vi "VI Tree.vi"   [LabVIEW 2012, in "Agilent ESG Series.lvlib"]
doc: "This is the instrument driver for the Hewlett Packard ESG/ESG-D Series Signal Generator. The VI Tree displays all the user-callable VIs of the instrument driver in an organized table.\n\n\nThis VI Tree contains all of the VI's in the LabVIEW template driver. These VI's are intended to be used as starting points for creating your own driver VIs for a particular instrument."
uses:
  <instrlib>/Agilent ESG Series/Agilent ESG Series.lvlib
panel:
  # "(c) 2005 - 2013 National Instruments.  ALL RIGHTS RESERVED."
  # "SEE DIAGRAM\nFOR VI TREE."
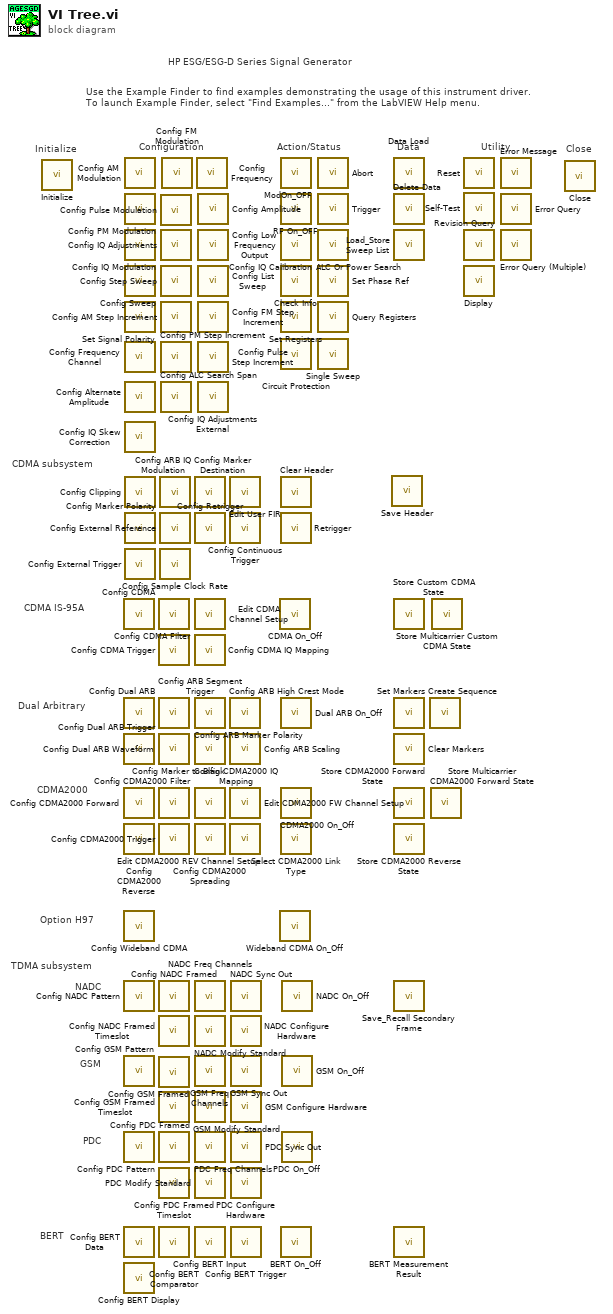
[diagram p0: block diagram]
diagram:
  # "HP ESG/ESG-D Series Signal Generator"
  # "CDMA2000"
  # "TDMA subsystem"
  # "CDMA subsystem"
  # "BERT"
  # "Option H97"
  # "Dual Arbitrary"
  # "CDMA IS-95A"
  # "PDC"
  # "GSM"
  # "NADC"
  # "Use the Example Finder to find examples demonstrating the usage of this instrument driver.\nTo launch Example Finder, select \"Find Examples...\" from the LabVIEW Help menu."
  # "Configuration"
  # "Utility"
  # "Data"
  # "Action/Status"
  # "Close"
  # "Initialize"
  n1 = call <instrlib>:"Initialize.vi"() -> ()  [unwired: 14 in, 2 out]
  n2 = call <instrlib>:"Config CDMA.vi"() -> ()  [unwired: 18 in, 2 out]
  n3 = call <instrlib>:"Config Dual ARB.vi"() -> ()  [unwired: 14 in, 2 out]
  n4 = call <instrlib>:"Config Dual ARB Trigger.vi"() -> ()  [unwired: 14 in, 2 out]
  n5 = call <instrlib>:"Config CDMA2000 Forward.vi"() -> ()  [unwired: 18 in, 2 out]
  n6 = call <instrlib>:"Config CDMA2000 Reverse.vi"() -> ()  [unwired: 18 in, 2 out]
  n7 = call <instrlib>:"Config Wideband CDMA.vi"() -> ()  [unwired: 14 in, 2 out]
  n8 = call <instrlib>:"Config NADC Pattern.vi"() -> ()  [unwired: 14 in, 2 out]
  n9 = call <instrlib>:"Config GSM Pattern.vi"() -> ()  [unwired: 14 in, 2 out]
  n10 = call <instrlib>:"Config PDC Pattern.vi"() -> ()  [unwired: 14 in, 2 out]
  n11 = call <instrlib>:"Config BERT Data.vi"() -> ()  [unwired: 18 in, 2 out]
  n12 = call <instrlib>:"Config BERT Display.vi"() -> ()  [unwired: 10 in, 2 out]
  n13 = call <instrlib>:"Config AM Modulation.vi"() -> ()  [unwired: 18 in, 2 out]
  n14 = call <instrlib>:"Config PM Modulation.vi"() -> ()  [unwired: 18 in, 2 out]
  n15 = call <instrlib>:"Config IQ Modulation.vi"() -> ()  [unwired: 14 in, 2 out]
  n16 = call <instrlib>:"Config Sweep.vi"() -> ()  [unwired: 18 in, 2 out]
  n17 = call <instrlib>:"Set Signal Polarity.vi"() -> ()  [unwired: 10 in, 2 out]
  n18 = call <instrlib>:"Config Frequency Channel.vi"() -> ()  [unwired: 14 in, 2 out]
  n19 = call <instrlib>:"Config Alternate Amplitude.vi"() -> ()  [unwired: 18 in, 2 out]
  n20 = call <instrlib>:"Config IQ Skew Correction.vi"() -> ()  [unwired: 14 in, 2 out]
  n21 = call <instrlib>:"Config Clipping.vi"() -> ()  [unwired: 18 in, 2 out]
  n22 = call <instrlib>:"Config Marker Polarity.vi"() -> ()  [unwired: 18 in, 2 out]
  n23 = call <instrlib>:"Config External Trigger.vi"() -> ()  [unwired: 14 in, 2 out]
  n24 = call <instrlib>:"Config CDMA Filter.vi"() -> ()  [unwired: 14 in, 2 out]
  n25 = call <instrlib>:"Config CDMA Trigger.vi"() -> ()  [unwired: 14 in, 2 out]
  n26 = call <instrlib>:"Config ARB Segment Trigger.vi"() -> ()  [unwired: 14 in, 2 out]
  n27 = call <instrlib>:"Config Dual ARB Waveform.vi"() -> ()  [unwired: 18 in, 2 out]
  n28 = call <instrlib>:"Config CDMA2000 Filter.vi"() -> ()  [unwired: 14 in, 2 out]
  n29 = call <instrlib>:"Config CDMA2000 Trigger.vi"() -> ()  [unwired: 14 in, 2 out]
  n30 = call <instrlib>:"Config NADC Framed.vi"() -> ()  [unwired: 14 in, 2 out]
  n31 = call <instrlib>:"Config NADC Framed Timeslot.vi"() -> ()  [unwired: 14 in, 2 out]
  n32 = call <instrlib>:"Config GSM Framed.vi"() -> ()  [unwired: 14 in, 2 out]
  n33 = call <instrlib>:"Config GSM Framed Timeslot.vi"() -> ()  [unwired: 18 in, 2 out]
  n34 = call <instrlib>:"Config PDC Framed.vi"() -> ()  [unwired: 14 in, 2 out]
  n35 = call <instrlib>:"Config PDC Framed Timeslot.vi"() -> ()  [unwired: 14 in, 2 out]
  n36 = call <instrlib>:"Config BERT Comparator.vi"() -> ()  [unwired: 10 in, 2 out]
  n37 = call <instrlib>:"Config ARB IQ Modulation.vi"() -> ()  [unwired: 14 in, 2 out]
  n38 = call <instrlib>:"Config External Reference.vi"() -> ()  [unwired: 18 in, 2 out]
  n39 = call <instrlib>:"Config Sample Clock Rate.vi"() -> ()  [unwired: 14 in, 2 out]
  n40 = call <instrlib>:"Config Pulse Modulation.vi"() -> ()  [unwired: 14 in, 2 out]
  n41 = call <instrlib>:"Config IQ Adjustments.vi"() -> ()  [unwired: 14 in, 2 out]
  n42 = call <instrlib>:"Config Step Sweep.vi"() -> ()  [unwired: 14 in, 2 out]
  n43 = call <instrlib>:"Config AM Step Increment.vi"() -> ()  [unwired: 14 in, 2 out]
  n44 = call <instrlib>:"Config PM Step Increment.vi"() -> ()  [unwired: 14 in, 2 out]
  n45 = call <instrlib>:"Config ALC Search Span.vi"() -> ()  [unwired: 18 in, 2 out]
  n46 = call <instrlib>:"Config FM Modulation.vi"() -> ()  [unwired: 18 in, 2 out]
  n47 = call <instrlib>:"Config Marker Destination.vi"() -> ()  [unwired: 18 in, 2 out]
  n48 = call <instrlib>:"Config Retrigger.vi"() -> ()  [unwired: 14 in, 2 out]
  n49 = call <instrlib>:"Edit CDMA Channel Setup.vi"() -> ()  [unwired: 14 in, 2 out]
  n50 = call <instrlib>:"Config CDMA IQ Mapping.vi"() -> ()  [unwired: 14 in, 2 out]
  n51 = call <instrlib>:"Config ARB Marker Polarity.vi"() -> ()  [unwired: 14 in, 2 out]
  n52 = call <instrlib>:"Config Marker to Blank.vi"() -> ()  [unwired: 14 in, 2 out]
  n53 = call <instrlib>:"Config CDMA2000 IQ Mapping.vi"() -> ()  [unwired: 14 in, 2 out]
  n54 = call <instrlib>:"Config CDMA2000 Spreading.vi"() -> ()  [unwired: 14 in, 2 out]
  n55 = call <instrlib>:"NADC Freq Channels.vi"() -> ()  [unwired: 10 in, 2 out]
  n56 = call <instrlib>:"NADC Modify Standard.vi"() -> ()  [unwired: 14 in, 2 out]
  n57 = call <instrlib>:"GSM Freq Channels.vi"() -> ()  [unwired: 10 in, 2 out]
  n58 = call <instrlib>:"GSM Modify Standard.vi"() -> ()  [unwired: 14 in, 2 out]
  n59 = call <instrlib>:"PDC Freq Channels.vi"() -> ()  [unwired: 10 in, 2 out]
  n60 = call <instrlib>:"PDC Modify Standard.vi"() -> ()  [unwired: 14 in, 2 out]
  n61 = call <instrlib>:"Config BERT Input.vi"() -> ()  [unwired: 14 in, 2 out]
  n62 = call <instrlib>:"Config Frequency.vi"() -> ()  [unwired: 14 in, 2 out]
  n63 = call <instrlib>:"Config Amplitude.vi"() -> ()  [unwired: 14 in, 2 out]
  n64 = call <instrlib>:"Config Low Frequency Output.vi"() -> ()  [unwired: 14 in, 2 out]
  n65 = call <instrlib>:"Config List Sweep.vi"() -> ()  [unwired: 14 in, 2 out]
  n66 = call <instrlib>:"Config FM Step Increment.vi"() -> ()  [unwired: 14 in, 2 out]
  n67 = call <instrlib>:"Config Pulse Step Increment.vi"() -> ()  [unwired: 14 in, 2 out]
  n68 = call <instrlib>:"Config IQ Adjustments External.vi"() -> ()  [unwired: 14 in, 2 out]
  n69 = call <instrlib>:"Edit User FIR.vi"() -> ()  [unwired: 14 in, 2 out]
  n70 = call <instrlib>:"Config Continuous Trigger.vi"() -> ()  [unwired: 14 in, 2 out]
  n71 = call <instrlib>:"Config ARB High Crest Mode.vi"() -> ()  [unwired: 14 in, 2 out]
  n72 = call <instrlib>:"Config ARB Scaling.vi"() -> ()  [unwired: 14 in, 2 out]
  n73 = call <instrlib>:"Edit CDMA2000 FW Channel Setup.vi"() -> ()  [unwired: 18 in, 2 out]
  n74 = call <instrlib>:"Edit CDMA2000 REV Channel Setup.vi"() -> ()  [unwired: 18 in, 2 out]
  n75 = call <instrlib>:"NADC Sync Out.vi"() -> ()  [unwired: 10 in, 2 out]
  n76 = call <instrlib>:"NADC Configure Hardware.vi"() -> ()  [unwired: 14 in, 2 out]
  n77 = call <instrlib>:"GSM Sync Out.vi"() -> ()  [unwired: 10 in, 2 out]
  n78 = call <instrlib>:"GSM Configure Hardware.vi"() -> ()  [unwired: 14 in, 2 out]
  n79 = call <instrlib>:"PDC Sync Out.vi"() -> ()  [unwired: 10 in, 2 out]
  n80 = call <instrlib>:"PDC Configure Hardware.vi"() -> ()  [unwired: 14 in, 2 out]
  n81 = call <instrlib>:"Config BERT Trigger.vi"() -> ()  [unwired: 10 in, 2 out]
  n82 = call <instrlib>:"CDMA On_Off.vi"() -> ()  [unwired: 14 in, 2 out]
  n83 = call <instrlib>:"Wideband CDMA On_Off.vi"() -> ()  [unwired: 14 in, 2 out]
  n84 = call <instrlib>:"ModOn_OFF.vi"() -> ()  [unwired: 14 in, 2 out]
  n85 = call <instrlib>:"RF On_OFF.vi"() -> ()  [unwired: 14 in, 2 out]
  n86 = call <instrlib>:"Config IQ Calibration.vi"() -> ()  [unwired: 14 in, 2 out]
  n87 = call <instrlib>:"Check Info.vi"() -> ()  [unwired: 13 in, 3 out]
  n88 = call <instrlib>:"Set Registers.vi"() -> ()  [unwired: 14 in, 2 out]
  n89 = call <instrlib>:"Circuit Protection.vi"() -> ()  [unwired: 14 in, 2 out]
  n90 = call <instrlib>:"Clear Header.vi"() -> ()  [unwired: 14 in, 2 out]
  n91 = call <instrlib>:"Retrigger.vi"() -> ()  [unwired: 14 in, 2 out]
  n92 = call <instrlib>:"Dual ARB On_Off.vi"() -> ()  [unwired: 14 in, 2 out]
  n93 = call <instrlib>:"CDMA2000 On_Off.vi"() -> ()  [unwired: 14 in, 2 out]
  n94 = call <instrlib>:"Select CDMA2000 Link Type.vi"() -> ()  [unwired: 14 in, 2 out]
  n95 = call <instrlib>:"BERT On_Off.vi"() -> ()  [unwired: 10 in, 2 out]
  n96 = call <instrlib>:"NADC On_Off.vi"() -> ()  [unwired: 14 in, 2 out]
  n97 = call <instrlib>:"GSM On_Off.vi"() -> ()  [unwired: 10 in, 2 out]
  n98 = call <instrlib>:"PDC On_Off.vi"() -> ()  [unwired: 10 in, 2 out]
  n99 = call <instrlib>:"Abort.vi"() -> ()  [unwired: 14 in, 2 out]
  n100 = call <instrlib>:"Trigger.vi"() -> ()  [unwired: 14 in, 2 out]
  n101 = call <instrlib>:"ALC Or Power Search.vi"() -> ()  [unwired: 14 in, 2 out]
  n102 = call <instrlib>:"Set Phase Ref.vi"() -> ()  [unwired: 14 in, 2 out]
  n103 = call <instrlib>:"Query Registers.vi"() -> ()  [unwired: 13 in, 3 out]
  n104 = call <instrlib>:"Single Sweep.vi"() -> ()  [unwired: 14 in, 2 out]
  n105 = call <instrlib>:"Save Header.vi"() -> ()  [unwired: 14 in, 2 out]
  n106 = call <instrlib>:"Data Load.vi"() -> ()  [unwired: 13 in, 3 out]
  n107 = call <instrlib>:"Delete Data.vi"() -> ()  [unwired: 14 in, 2 out]
  n108 = call <instrlib>:"Load_Store Sweep List.vi"() -> ()  [unwired: 14 in, 2 out]
  n109 = call <instrlib>:"Store Custom CDMA State.vi"() -> ()  [unwired: 14 in, 2 out]
  n110 = call <instrlib>:"Set Markers.vi"() -> ()  [unwired: 18 in, 2 out]
  n111 = call <instrlib>:"Clear Markers.vi"() -> ()  [unwired: 18 in, 2 out]
  n112 = call <instrlib>:"Store CDMA2000 Forward State.vi"() -> ()  [unwired: 14 in, 2 out]
  n113 = call <instrlib>:"Store CDMA2000 Reverse State.vi"() -> ()  [unwired: 14 in, 2 out]
  n114 = call <instrlib>:"Save_Recall Secondary Frame.vi"() -> ()  [unwired: 14 in, 2 out]
  n115 = call <instrlib>:"BERT Measurement Result.vi"() -> ()  [unwired: 13 in, 3 out]
  n116 = call <instrlib>:"Create Sequence.vi"() -> ()  [unwired: 18 in, 2 out]
  n117 = call <instrlib>:"Store Multicarrier CDMA2000 Forward State.vi"() -> ()  [unwired: 14 in, 2 out]
  n118 = call <instrlib>:"Store Multicarrier Custom CDMA State.vi"() -> ()  [unwired: 14 in, 2 out]
  n119 = call <instrlib>:"Reset.vi"() -> ()  [unwired: 14 in, 2 out]
  n120 = call <instrlib>:"Self-Test.vi"() -> ()  [unwired: 12 in, 4 out]
  n121 = call <instrlib>:"Revision Query.vi"() -> ()  [unwired: 12 in, 4 out]
  n122 = call <instrlib>:"Display.vi"() -> ()  [unwired: 10 in, 2 out]
  n123 = call <instrlib>:"Error Message.vi"() -> ()  [unwired: 11 in, 5 out]
  n124 = call <instrlib>:"Error Query.vi"() -> ()  [unwired: 12 in, 4 out]
  n125 = call <instrlib>:"Error Query (Multiple).vi"() -> ()  [unwired: 12 in, 4 out]
  n126 = call <instrlib>:"Close.vi"() -> ()  [unwired: 15 in, 1 out]
